vi "Configure TDMS DAQ.vi"(4 "Batch Size":i32, 6 "Thread Count":i32, 8 "error in (no error)":errorcluster, 10 "Path":path, 11 "TDMS DAQ in":refnum<class "TDMS DAQ.lvclass">) -> (0 "error out":errorcluster, 3 "TDMS DAQ out":refnum<class "TDMS DAQ.lvclass">)   [LabVIEW 2020, in "TDMS DAQ.lvlib" / "TDMS DAQ.lvclass"]
uses:
  TDMS DAQ.lvclass
  Configure TDMS DAQ.ctl
  Helper Loop Message.ctl
  Helper Loop Type.ctl
  TDMS DAQ.lvclass/TDMS DAQ.ctl
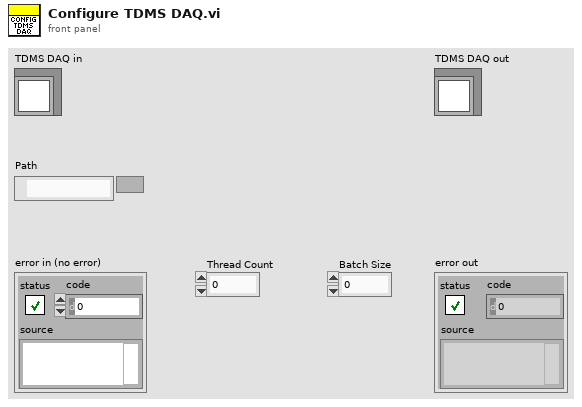
[diagram p1: front panel]
types:
  T1 = typedef "TDMS DAQ.lvlib/TDMS DAQ.lvclass/Helper Loop Type.ctl" = enum16{"Configure", "Start", "Do", "Stop", "Clean", "Close"}
  T2 = typedef "TDMS DAQ.lvlib/TDMS DAQ.lvclass/Helper Loop Message.ctl" = cluster{"Type":T1, "Payload":variant}
  T3 = typedef "TDMS DAQ.lvlib/TDMS DAQ.lvclass/Configure TDMS DAQ.ctl" = cluster{"Path":path, "Thread Count":i32, "Batch Size":i32}
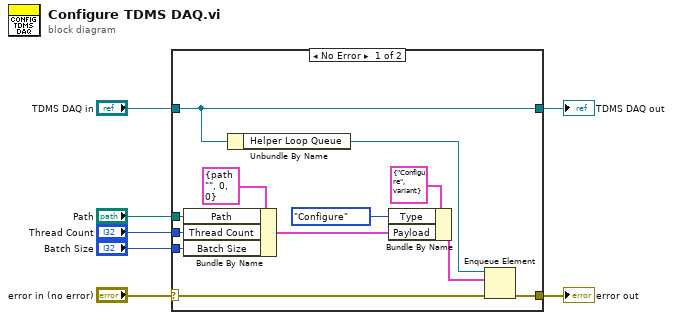
[diagram p0: block diagram]
diagram:
  n1 = case shown="No Error" "error in (no error)" {
    selector: "error in (no error)" -> [w17 w21]
    tunnel: [w16 w21] -> w6
    tunnel: [w19 w20] -> w4
    tunnel: "TDMS DAQ in" -> [w19 w20]
    tunnel: "Path" -> [w15 _]
    tunnel: "Thread Count" -> [w14 _]
    tunnel: "Batch Size" -> [w13 _]
    frame No Error {
      n2 = Bundle By Name(cluster=T3 {"Path"=path "", "Thread Count"=0, "Batch Size"=0} ("output cluster"), "Path"=w15, "Thread Count"=w14, "Batch Size"=w13) -> (w9:T3)
      n3 = Unbundle By Name(w19) -> ("Helper Loop Queue"=w18:refnum<queue>)
      n4 = Bundle By Name(cluster=T2 {"Type"=enum."Configure", "Payload"=variant} ("element"), "Type"=Helper_Loop_Type."Configure", "Payload"=w9) -> (w10:T2)
      n5 = Enqueue Element(queue=w18, element=w10, error in (no error)=w17) -> (error out=w16:errorcluster)  [unwired: 1 in, 2 out]
    }
    frame Error {
    }
  }
  "error out" <- w6
  "TDMS DAQ out" <- w4
